vi "FTDI - Float to Byte.vi"(11 "Float":sgl) -> (3 "Byte":u8[](array[numeric]))   [LabVIEW 2019]
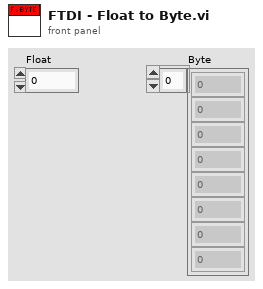
[diagram p1: front panel]
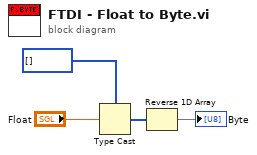
[diagram p0: block diagram]
diagram:
  n1 = Type Cast(type=u8[] [], x="Float") -> (*(type *) &x=w2:u8[])
  n2 = Reverse 1D Array(array=w2) -> (reversed array=→"Byte":u8[])
